vi "Send.vi"(0 "handles cluster in":T1 caption="ハンドルクラスター入力", 11 "error in (no error)":errorcluster caption="エラー入力（エラーなし）", 12 "timeout in ms (10000)":i32=10000 caption="タイムアウト（ms）（10000）") -> (4 "handles cluster out":T1 caption="ハンドルクラスター出力", 15 "error out":errorcluster caption="エラー出力")   [LabVIEW 2015]
doc: "ハンドルクラスター入力に配線したハンドルで設定した構成を使用してEメールを送信します。\n※ 組み込みの「SMTP EメールVI」の「送信」VIにある「無効な受信者」は実装していません。"
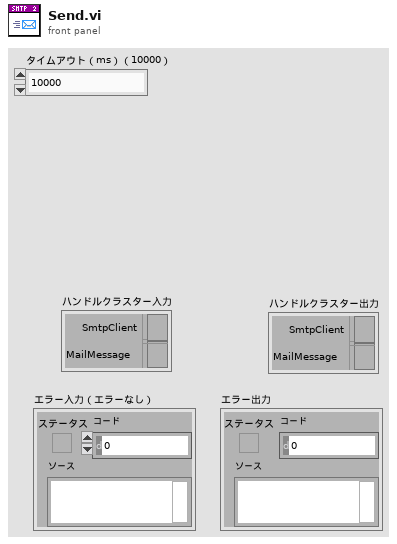
[diagram p1: front panel]
types:
  T1 = cluster{"SmtpClient":refnum<k24>, "MailMessage":refnum<k24>}
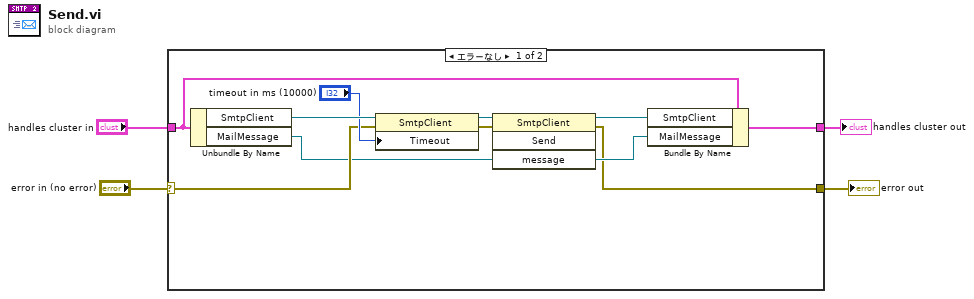
[diagram p0: block diagram]
diagram:
  n1 = case shown="エラーなし" "error in (no error)" {
    selector: "error in (no error)" -> [w11 w16]
    tunnel: [w6 w16] -> w3
    tunnel: "handles cluster in" -> [w8 w15]
    tunnel: [w5 w15] -> w1
    frame No Error {
      n2 = Unbundle By Name(w8) -> ("SmtpClient"=w14:refnum<k24>, "MailMessage"=w7:refnum<k24>)
      n3 = property class="SmtpClient"(reference=w14, error in=w11, "Timeout"="timeout in ms (10000)") -> (reference out=w12:refnum<k24>, error out=w10:errorcluster)
      n4 = invoke class="SmtpClient" method="Send"(reference=w12, error in=w10, "message"=w7) -> (reference out=w9:refnum<k24>, error out=w6:errorcluster)  [unwired: 1 in, 2 out]
      n5 = Bundle By Name(cluster=w8, "SmtpClient"=w9, "MailMessage"=w7) -> (w5:T1)
    }
    frame Error {
    }
  }
  "handles cluster out" <- w1
  "error out" <- w3
